vi "CRYHarmonics list editor.vi"(10 "Checkoffs":bool[](array[boolean]), 11 "Items":string[](array[string])) -> (1 "Checkoffs out":bool[](array[boolean]), 2 "Symbols out":i32[](array[numeric]), 3 "Items out":string[](array[string]))   [LabVIEW 2013]
panel:
  in  "cont":bool
  in  "ok":bool
  in  "cancel":bool
  in  "to button":bool
  in  "remove":bool
  in  "har2":dbl=5.0 format="%.2f"
  in  "har1":dbl=2.0 format="%.2f"
  in  "add":bool
  in  "Harmonics":i32(listbox) caption="谐波"
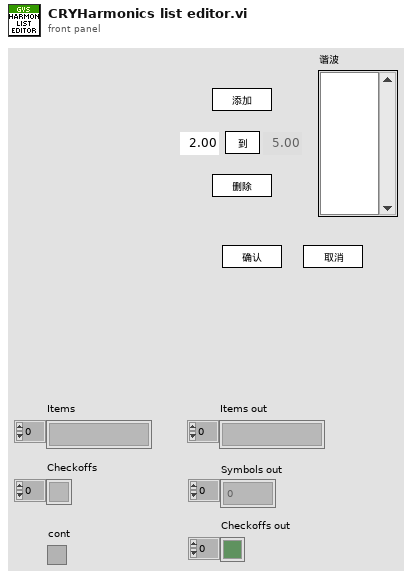
[diagram p1: front panel]
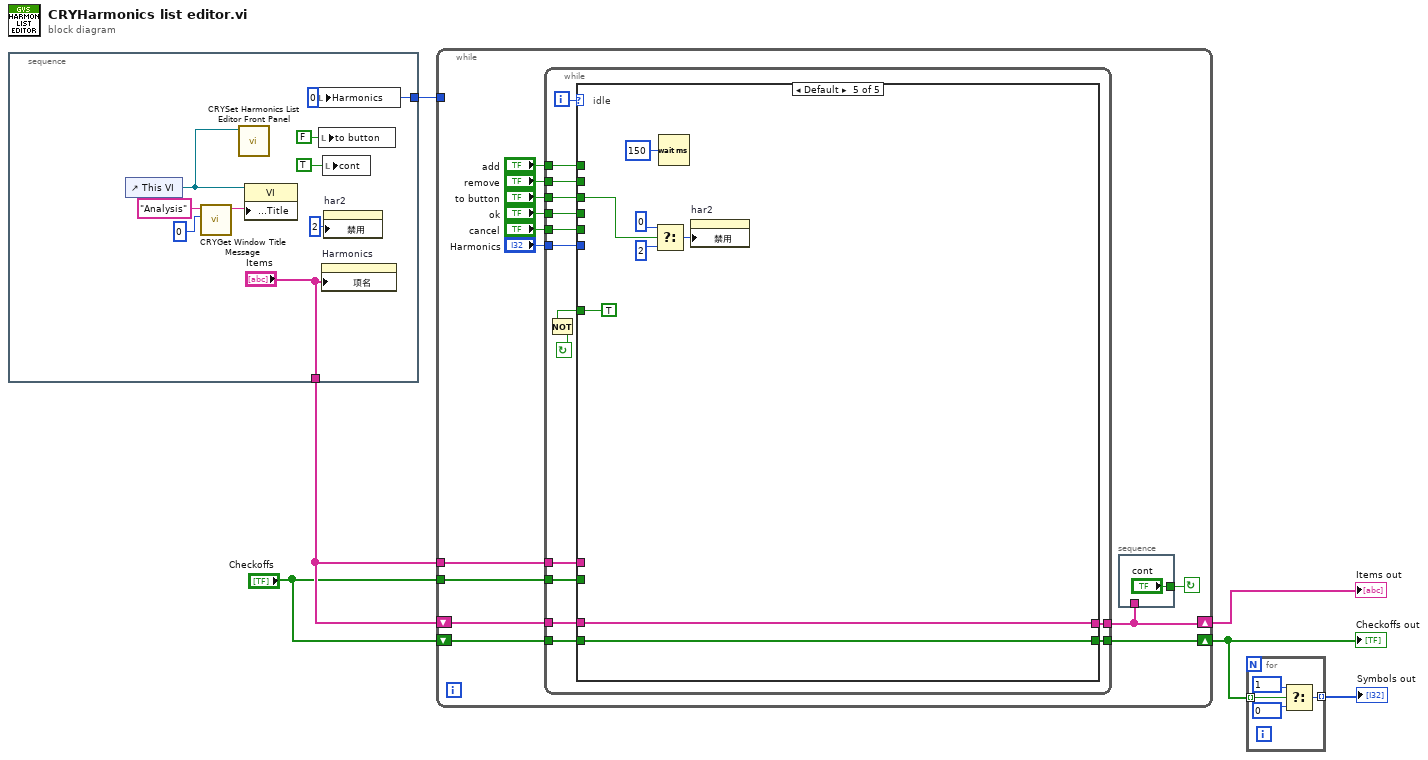
[diagram p0: block diagram]
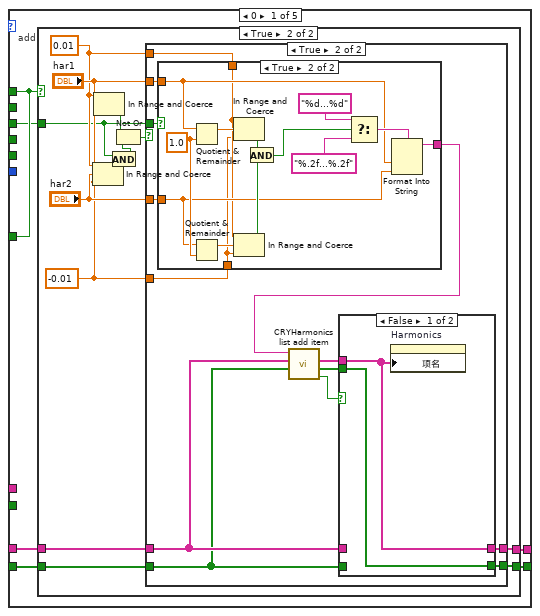
[diagram p2: hidden frame]
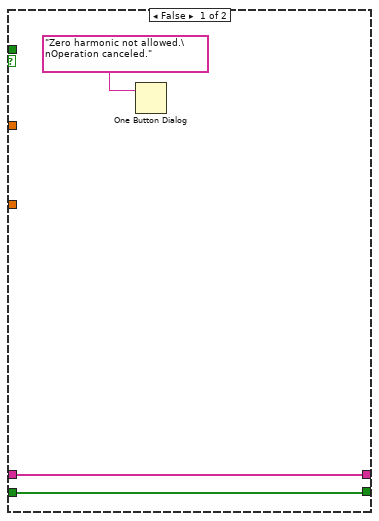
[diagram p4: hidden frame]
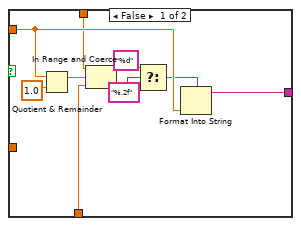
[diagram p5: hidden frame]
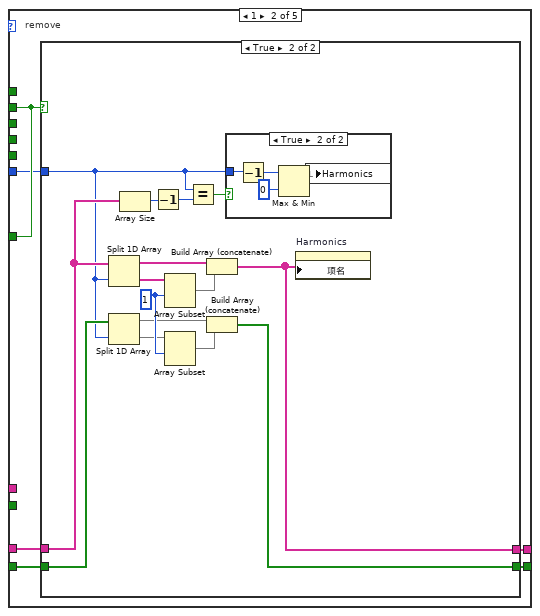
[diagram p7: hidden frame]
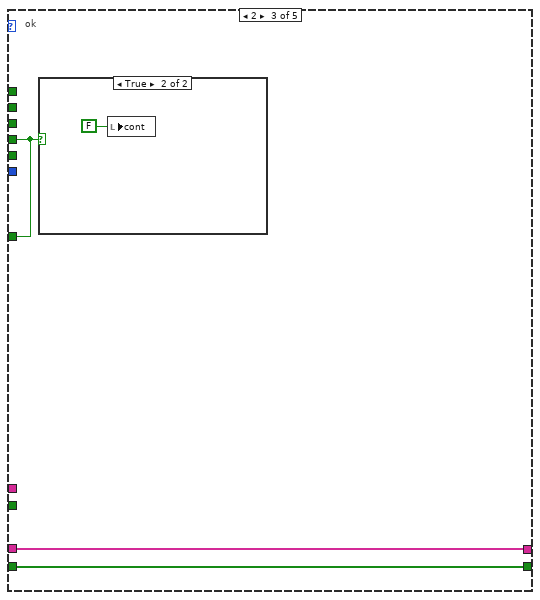
[diagram p10: hidden frame]
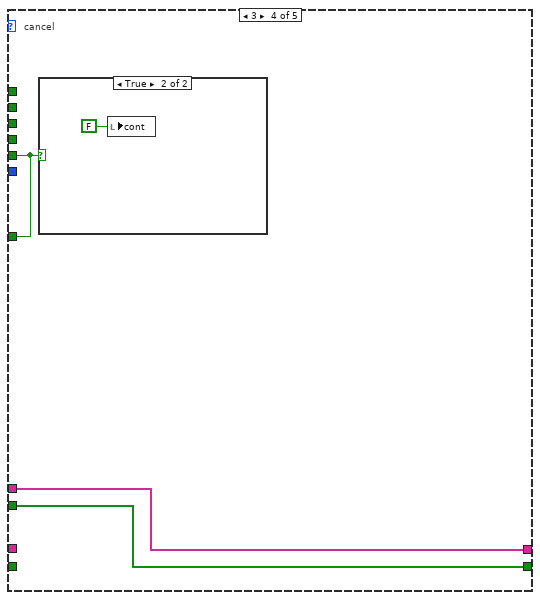
[diagram p12: hidden frame]
diagram:
  n1 = stacked-sequence {
    tunnel: [w15] -> w6
    tunnel: ["Items"] -> w2
    frame #0 {
      w15 = 0 ("Harmonics")
      n2 = control-ref of="This VI"() -> (w10:refnum<vi>)
      n3 = call "CRYGet Window Title Message.vi"("No"=0 ("Error No"), "Kind"="Analysis") -> ("Multibyte String"=w7:string)  [unwired: 4 in, 5 out]
      n4 = call "CRYSet Harmonics List Editor Front Panel.vi"("Vi Ref"=w10) -> ()  [unwired: 11 in]
      n5 = property class="VI"(reference=w10, "Front Panel.Title"=w7) -> ()  [unwired: 1 in, 2 out]
      n6 = local write "Harmonics"(w15) -> ()
      n7 = local write "to button"(FALSE ("to button")) -> ()
      n8 = property on="Harmonics" class="LstBox (strict)"("项名"="Items") -> ()  [unwired: 2 in, 2 out]
      n9 = local write "cont"(TRUE ("cont")) -> ()
      n10 = property on="har2" class="DigNum (strict)"("禁用"=u8 2 ("Write Attribute")) -> ()  [unwired: 2 in, 2 out]
    }
  }
  n11 = while {
    tunnel: "Checkoffs" -> [w18]
    tunnel: w2 -> [w19]
    shift-left: "Checkoffs" -> [w25]
    shift-right: [w24] -> w4
    shift-left: w2 -> [w26]
    shift-right: [w16] -> w5
    tunnel: w6 -> [_]
    stop <- w17 continue-if-true
    n12 = while {
      tunnel: w18 -> [w29]
      tunnel: w19 -> [w30]
      tunnel: "cancel" -> [w31]
      tunnel: "ok" -> [w32]
      tunnel: "Harmonics" -> [w33]
      tunnel: "remove" -> [w34]
      tunnel: [w35] -> w16
      tunnel: [w36] -> w24
      tunnel: w25 -> [w37]
      tunnel: w26 -> [w38]
      tunnel: "to button" -> [w39]
      tunnel: "add" -> [w40]
      i -> [w41]
      stop <- w43 continue-if-true
      n13 = case shown="Default" w41 {
        tunnel: [w49 w114 w138 w142 TRUE] -> w42
        tunnel: w40 -> [w49 _ _ _ _]
        tunnel: w39 -> [w48 _ _ _ w147]
        tunnel: w38 -> [w47 w113 w137 _ w151]
        tunnel: w37 -> [w46 w112 w136 _ w150]
        tunnel: [w45 w109 w136 w140 w150] -> w36
        tunnel: [w44 w110 w137 w141 w151] -> w35
        tunnel: w34 -> [_ w114 _ _ _]
        tunnel: w33 -> [_ w111 _ _ _]
        tunnel: w32 -> [_ _ w138 _ _]
        tunnel: w31 -> [_ _ _ w142 _]
        tunnel: w30 -> [_ _ _ w141 _]
        tunnel: w29 -> [_ _ _ w140 _]
        frame 0 {
          # "add"
          n14 = case shown="True" w49 {
            tunnel: w48 -> [_ w54]
            tunnel: w47 -> [w51 w62]
            tunnel: w46 -> [w50 w61]
            tunnel: [w50 w63] -> w45
            tunnel: [w51 w64] -> w44
            frame False {
            }
            frame True {
              w58 = -0.01
              w57 = 0.01
              n15 = In Range and Coerce(upper limit=w57, x="har2", lower limit=w58) -> (In Range?=w55:bool)  [unwired: 1 out]
              n16 = In Range and Coerce(upper limit=w57, x="har1", lower limit=w58) -> (In Range?=w56:bool)  [unwired: 1 out]
              n17 = And(x=w54, y=w55) -> (x .and. y?=w53:bool)
              n18 = Not Or(1:w53, 2:w56) -> (0:w52:bool)
              n19 = case shown="True" w52 {
                tunnel: w54 -> [_ w80]
                tunnel: "har1" -> [_ w79]
                tunnel: "har2" -> [_ w78]
                tunnel: [w67 w74] -> w64
                tunnel: [w66 w73] -> w63
                tunnel: w62 -> [w67 w71]
                tunnel: w61 -> [w66 w70]
                tunnel: w57 -> [_ w69]
                tunnel: w58 -> [_ w68]
                frame False {
                  n20 = One Button Dialog(message="Zero harmonic not allowed.\nOperation canceled.") -> ()  [unwired: 2 out]
                }
                frame True {
                  n21 = case shown="True" w80 {
                    tunnel: w79 -> [w85 w100]
                    tunnel: [w83 w93] -> w77
                    tunnel: w78 -> [_ w94]
                    tunnel: w69 -> [w82 w92]
                    tunnel: w68 -> [w81 w91]
                    frame False {
                      n22 = Quotient & Remainder(x=w85, y=1.0) -> (x-y*floor(x/y)=w90:dbl)  [unwired: 1 out]
                      n23 = In Range and Coerce(upper limit=w82, x=w90, lower limit=w81) -> (In Range?=w88:bool)  [unwired: 1 out]
                      n24 = Select(t="%d", s=w88, f="%.2f") -> (s? t:f=w84:string)
                      n25 = Format Into String(format string=w84, w85) -> (resulting string=w83:string)  [unwired: 2 in, 1 out]
                    }
                    frame True {
                      w98 = 1.0
                      n26 = Quotient & Remainder(x=w100, y=w98) -> (x-y*floor(x/y)=w104:dbl)  [unwired: 1 out]
                      n27 = Quotient & Remainder(x=w94, y=w98) -> (x-y*floor(x/y)=w99:dbl)  [unwired: 1 out]
                      n28 = In Range and Coerce(upper limit=w92, x=w104, lower limit=w91) -> (In Range?=w97:bool)  [unwired: 1 out]
                      n29 = In Range and Coerce(upper limit=w92, x=w99, lower limit=w91) -> (In Range?=w96:bool)  [unwired: 1 out]
                      n30 = And(x=w97, y=w96) -> (x .and. y?=w95:bool)
                      n31 = Select(t="%d...%d", s=w95, f="%.2f...%.2f") -> (s? t:f=w101:string)
                      n32 = Format Into String(format string=w101, w100, w94) -> (resulting string=w93:string)  [unwired: 2 in, 1 out]
                    }
                  }
                  n33 = call "CRYHarmonics list add item.vi"("Checkoffs"=w70, "Items"=w71, "Candidate item"=w77) -> ("Cancel operation"=w75:bool, "Checkoffs out"=w72:bool[], "Items out"=w76:string[])  [unwired: 6 out]
                  n34 = case shown="False" w75 {
                    tunnel: w76 -> [w106 _]
                    tunnel: [w106 w108] -> w74
                    tunnel: [w105 w107] -> w73
                    tunnel: w72 -> [w105 _]
                    tunnel: w71 -> [_ w108]
                    tunnel: w70 -> [_ w107]
                    frame False {
                      n35 = property on="Harmonics" class="LstBox (strict)"("项名"=w106) -> ()  [unwired: 2 in, 2 out]
                    }
                    frame True {
                    }
                  }
                }
              }
            }
          }
        }
        frame 1 {
          # "remove"
          n36 = case shown="True" w114 {
            tunnel: w113 -> [w116 w121]
            tunnel: w112 -> [w115 w130]
            tunnel: w111 -> [_ w117]
            tunnel: [w116 w122] -> w110
            tunnel: [w115 w123] -> w109
            frame False {
            }
            frame True {
              w131 = 1 ("Array Index")
              n37 = Split 1D Array(array=w121, index=w117) -> (first subarray=w129:string[], second subarray=w128:string[])
              n38 = Split 1D Array(array=w130, index=w117) -> (first subarray=w127:bool[], second subarray=w126:bool[])
              n39 = Array Size(array=w121) -> (size(s)=w120:i32)
              n40 = Decrement(x=w120) -> (x-1=w119:i32)
              n41 = Array Subset(array=w128, index=w131) -> (w124:string[])  [unwired: 1 in]
              n42 = Array Subset(array=w126, index=w131) -> (w125:bool[])  [unwired: 1 in]
              n43 = Equal?(x=w117, y=w119) -> (x = y?=w118:bool)
              n44 = Build Array (concatenate)(w129, w124) -> (w122:string[])
              n45 = Build Array (concatenate)(w127, w125) -> (w123:bool[])
              n46 = case shown="True" w118 {
                tunnel: w117 -> [_ w135]
                frame False {
                }
                frame True {
                  n47 = Decrement(x=w135) -> (x-1=w134:i32)
                  n48 = Max & Min(x=w134, y=0) -> (max(x,y)=w132:i32)  [unwired: 1 out]
                  n49 = local write "Harmonics"(w132) -> ()
                }
              }
              n50 = property on="Harmonics" class="LstBox (strict)"("项名"=w122) -> ()  [unwired: 2 in, 2 out]
            }
          }
        }
        frame 2 {
          # "ok"
          n51 = case shown="True" w138 {
            frame False {
            }
            frame True {
              n52 = local write "cont"(FALSE ("cont")) -> ()
            }
          }
        }
        frame 3 {
          # "cancel"
          n53 = case shown="True" w142 {
            frame False {
            }
            frame True {
              n54 = local write "cont"(FALSE ("cont")) -> ()
            }
          }
        }
        frame Default {
          # "idle"
          n55 = Select(t=u8 0 ("Write Attribute"), s=w147, f=u8 2 ("Write Attribute")) -> (s? t:f=w144:u8)
          n56 = Wait (ms)(milliseconds to wait=u32 150) -> ()  [unwired: 1 out]
          n57 = property on="har2" class="DigNum (strict)"("禁用"=w144) -> ()  [unwired: 2 in, 2 out]
        }
      }
      n58 = Not(x=w42) -> (.not. x?=w43:bool)
    }
    n59 = stacked-sequence {
      tunnel: ["cont"] -> w17
      tunnel: w16 -> [_]
      frame #0 {
      }
    }
  }
  "Items out" <- w5
  "Checkoffs out" <- w4
  n60 = for {
    tunnel: w4 -> [w156] mode=indexing
    tunnel: [w155] -> w3 mode=indexing
    n61 = Select(t=1, s=w156, f=0) -> (s? t:f=w155:i32)
  }
  "Symbols out" <- w3
